vi "TLB Native Dynamic Events ver 0.08b.vi"() -> ()   [LabVIEW 2018]
uses:
  Labview Training Phase 2/Enum Controls/States for Action Engine.ctl
  Type def/TLB event states.ctl
  Type def/TLB MHL States.ctl
  <vilib>/Studica/Studica Toolkit/Background/I2C Channel.ctl
  <vilib>/Studica/Studica Toolkit/NavX/NavX.lvlib
  <vilib>/myRIO/Common/Instrument Driver Framework/myRIO v1.0/AI/typedefs/AI Channels Enum.ctl
  <vilib>/myRIO/Common/Instrument Driver Framework/myRIO v1.0/AI/typedefs/AI Channels List.ctl
  Type def/Type def.ctl
  <vilib>/Studica/Studica Blackhawk/Blackhawk.lvlib
  <vilib>/Studica/Studica Toolkit/Background/Mxp Selection.ctl
  <vilib>/Studica/Studica Toolkit/Background/DIO Channel.ctl
  <vilib>/NI_Real-Time Target Support.lvlib
  <vilib>/ptbypt/NI_PtbyPt.lvlib
  <vilib>/addons/control/pid/NI_PID_pid.lvlib
  Underlying VI's/Webcam FGV Low level ver/State control.ctl
  <vilib>/userdefined/High Color/IMAQdx.ctl
  <vilib>/addons/control/pid/pid.llb/PID (DBL).vi
panel:
  out "Speed and distance cluster":T1
  out "Output":dbl
  in  "SENSOR":bool
  out "Decision":i8
  out "Manual Zero Yaw":bool
  out "Displacement":T2
  out "Fused Heading":dbl
  in  "error in (no error)":errorcluster
  in  "RED LED State":enum16{"OFF", "ON", "BLINK"}(ring)
  in  "GREEN LED State":enum16{"OFF", "ON", "BLINK"}(ring)
  in  "Red LED":bool
  in  "Green LED":bool
  in  "NavX Zero Yaw":bool
  out "Input state":i8
  out "Waveform Chart 2":dbl(graph)
  out "Waveform Chart":dbl(graph)
  in  "STOP":bool
  out "DIO 0":bool
  out "DIO 1":bool
  out "Limit Switch Array":bool[](array[boolean])
  out "error out":errorcluster
  out "L/R average":fxp<+,64,64>
  out "Right Ultrasonic":fxp<+,64,16>
  out "Left Ultrasonic":fxp<+,64,16>
  out "Right IR Sensor":dbl
  out "Left IR Sensor":dbl
  out "Object detection count":T3
  out "Camera error":errorcluster
  in  "Servo Angle":u8(slide) scale=0.0..180.0
  in  "On/Off":bool
  out "Error":errorcluster
  out "element":T4
  out "Action Queue Items":i32
  out "State Logic Queue Items":i32
  out "Action Queues items":string[](array[string])=["Hardware reset", "Software reset", ""]
  out "State logic":T5=enum."Task 2"
  out "Action State":string
  out "Yaw":dbl
  # "TLB FRAMEWORK STATUS"
  # "Camera Status Loop"
  # "Test Programme written by Calvin Loke    Dated: 28 Aug 2019\nTest Programme revised by Dr Alex See   Dated 30 Aug 2019\n\nProgramme version:   TLB Native Dynamic Events ver 0.04b.vi"
  # "Problems now:\nYaw does not work when code is in last state mode\nSlow acceleration due to loop rate?"
  # "Motor Control Loop"
  # "NAVX Control Loop"
  # "Blackhawk status"
  # "Sensor data"
  # "System Health Status Update"
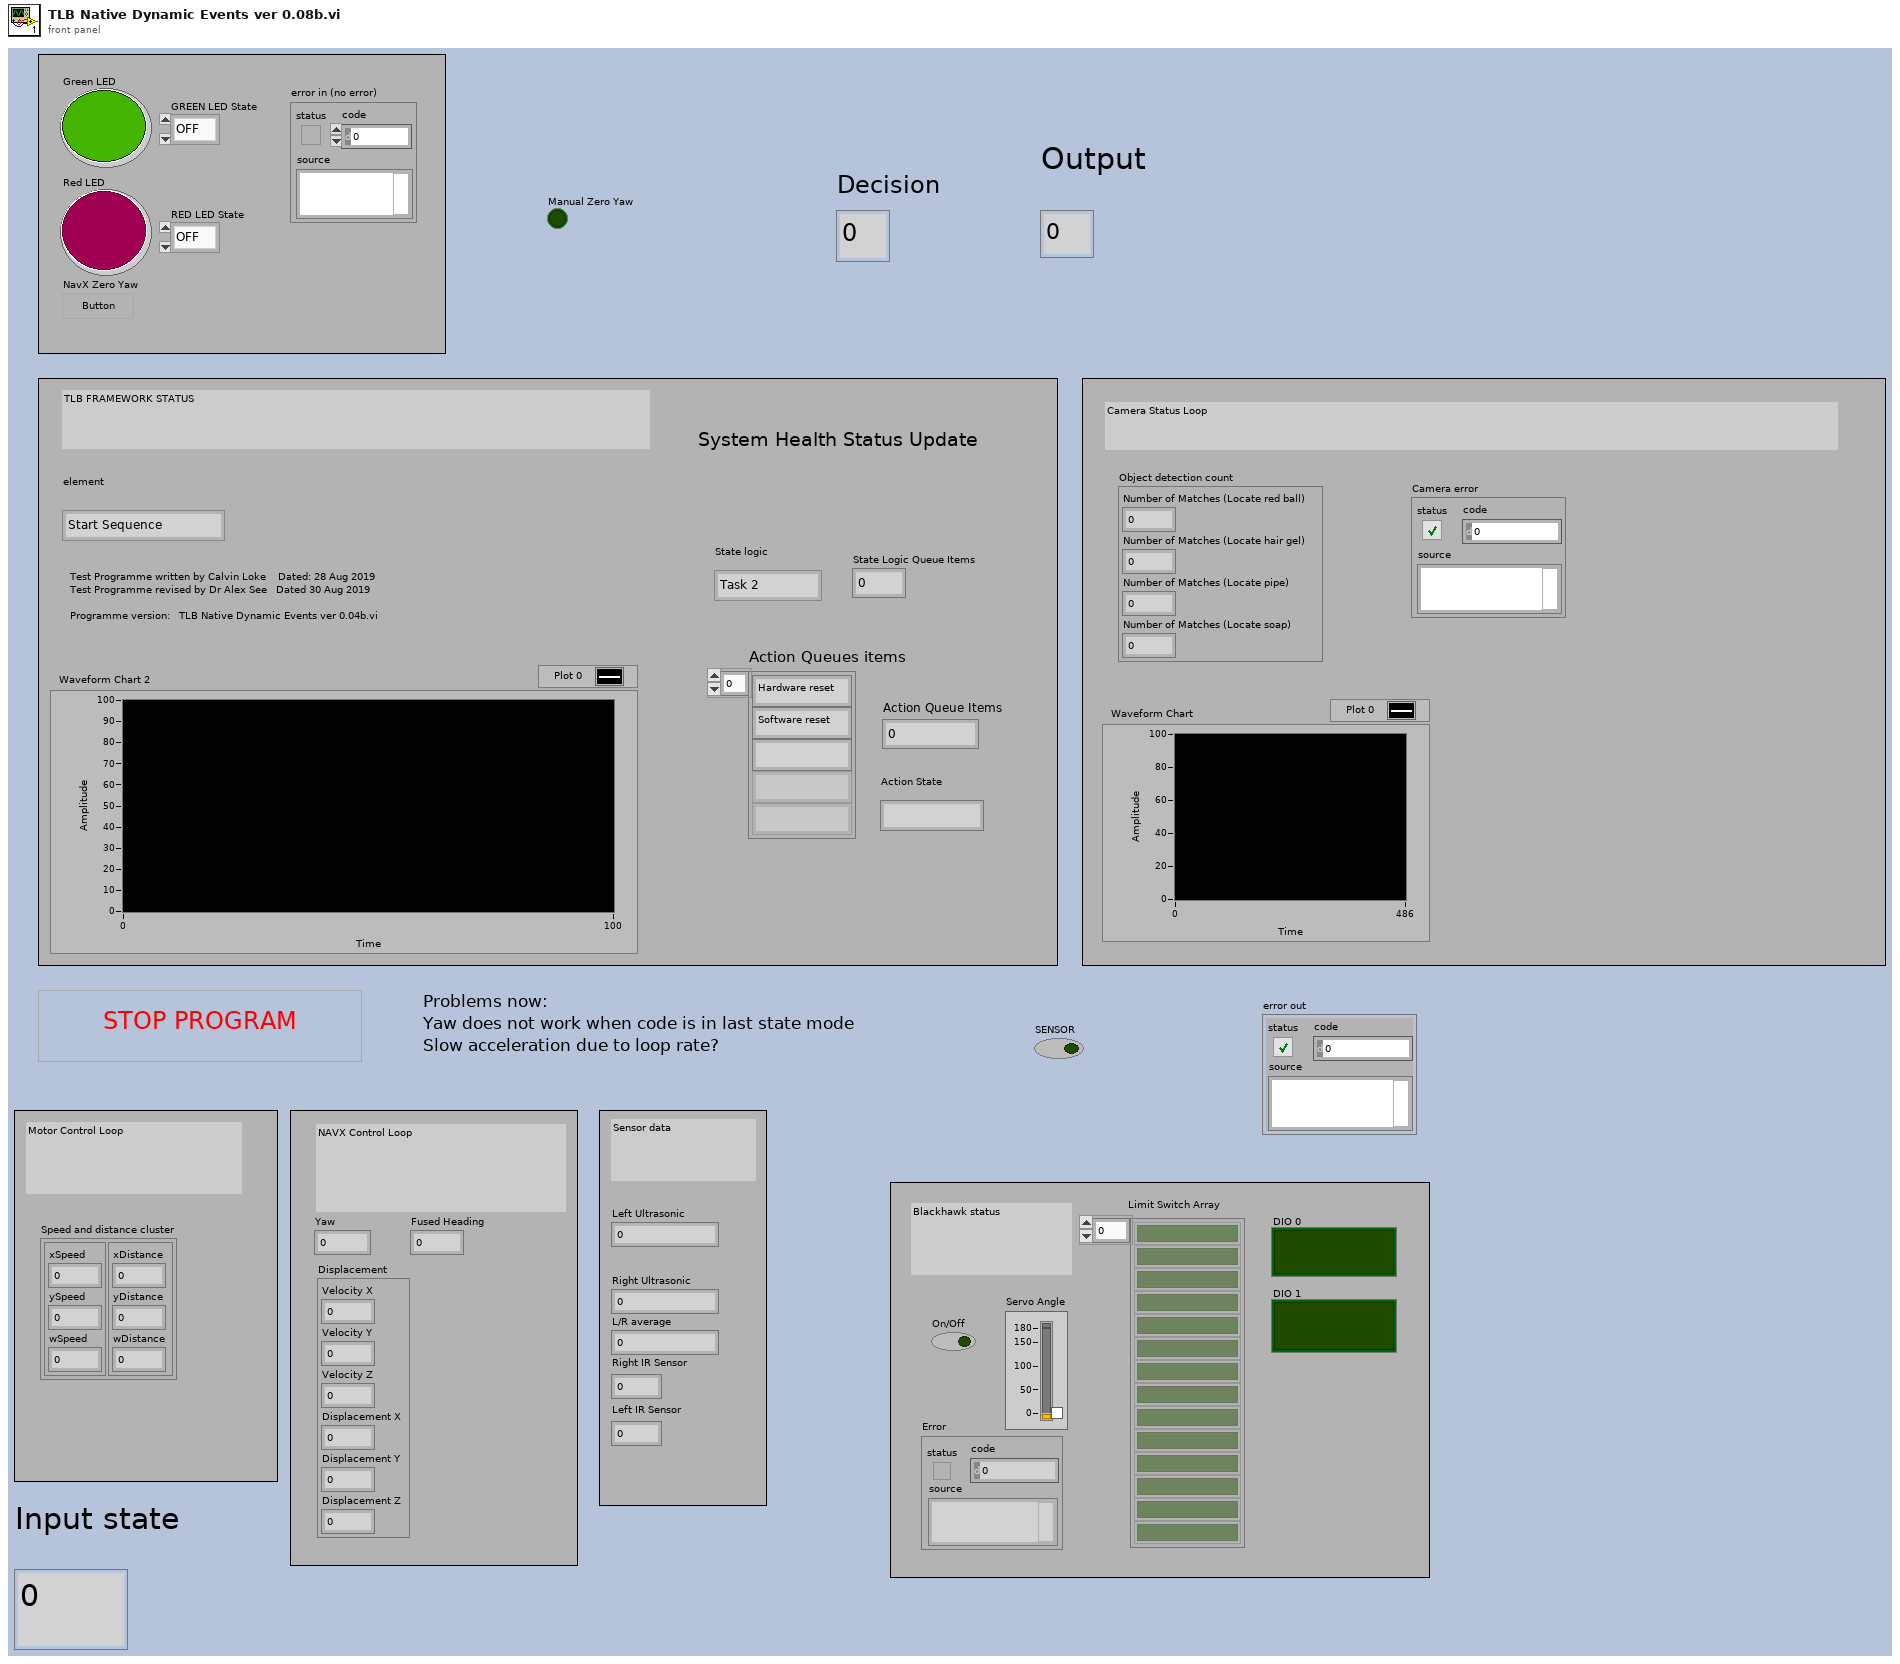
[diagram p1: front panel]
types:
  T1 = cluster{cluster{"xSpeed":dbl, "ySpeed":dbl, "wSpeed":dbl}, cluster{"xDistance":dbl, "yDistance":dbl, "wDistance":dbl}}
  T2 = cluster{"Velocity X":dbl, "Velocity Y":dbl, "Velocity Z":dbl, "Displacement X":dbl, "Displacement Y":dbl, "Displacement Z":dbl}
  T3 = cluster{"Number of Matches (Locate red ball)":i32, "Number of Matches (Locate hair gel)":i32, "Number of Matches (Locate pipe)":i32, "Number of Matches (Locate soap)":i32}
  T4 = typedef "TLB event states.ctl" = enum16{"Start Sequence", "Exit", "Start Task 1", "Start Task 2", "Start Task 3", "Start Task 4", "Camera vision", "Wall follow mode", "Idle", "Start Drive Straight"}
  T5 = typedef "TLB MHL States.ctl" = enum16{"None", "Startup", "Idle", "Processing", "Shutdown", "Reset", "Task 1", "Task 2", "Task 3", "Task 4", "Task 4a", "Task 4b", "Task 4c", "Task 4d", "Task 4e", "Task 4f", "Task 4g", "Task 4h", "Acquire image", "Wall follow mode", "Autodrive", "Autodrive a"}
  T6 = typedef "States for Action Engine.ctl" = enum16{"Initialize", "Write", "Read"}
  T7 = typedef "DIO Channel.ctl" = enum16{"Not Connected", "A/DIO1", "A/DIO2", "A/DIO3", "A/DIO4", "A/DIO5", "A/DIO6", "A/DIO7", "A/DIO13", "B/DIO1", "B/DIO2", "B/DIO3", "B/DIO4", "B/DIO5", "B/DIO6", "B/DIO7", "B/DIO13", "C/DIO0", "C/DIO1", "C/DIO2", "C/DIO3", "C/DIO4", "C/DIO5", "C/DIO6", "C/DIO7"}
  T8 = typedef "Type def.ctl" = cluster{"Front Ultrasonic Obstruct":bool, "Left Ultrasonic Obstruct":bool, "Right Ultrasonic Obstruct ":bool}
  T9 = typedef "I2C Channel.ctl" = enum16{"Not Connected", "A", "B"}
  T10 = enum16{"LAST STATE", "STOP", "FORWARD", "BACKWARD", "LEFT", "RIGHT", "RCW", "ACW", "INIT", "RESET ENCODERS"}
  T11 = cluster{"proportional gain (Kc)":dbl, "integral time (Ti, min)":dbl, "derivative time (Td, min)":dbl}
  T12 = typedef "State control.ctl" = enum16{"Initialise", "Start camera", "Continuous Acquisition ", "Stop camera", "Dispose all"}
  T13 = typedef "IMAQdx.ctl" = refnum<k21>
  T14 = typedef "Mxp Selection.ctl" = enum16{"MXP A", "MXP B"}
  T15 = enum16{"DISTANCE READ", "STOP", "FORWARD", "BACKWARD", "LEFT", "RIGHT", "RCW", "ACW", "INIT", "RESET ENCODERS"}
  T16 = typedef "AI Channels List.ctl" = T17[]
  T17 = typedef "AI Channels Enum.ctl" = enum16{"Not Connected", "AudioIn/Left", "AudioIn/Right", "C/AI0", "C/AI1", "A/AI0", "A/AI1", "A/AI2", "A/AI3", "A/AI4", "A/AI5", "A/AI6", "A/AI7", "B/AI0", "B/AI1", "B/AI2", "B/AI3", "B/AI4", "B/AI5", "B/AI6", "B/AI7", "AI/AI0", "AI/AI1", "AI/AI2", "AI/AI3", "A/AI0 (DIFF)", "A/AI1 (DIFF)", "A/AI2 (DIFF)", "A/AI3 (DIFF)", "B/AI0 (DIFF)", "B/AI1 (DIFF)", "B/AI2 (DIFF)", "B/AI3 (DIFF)"}
  T18 = cluster{"DIO Channel":T7, "FPGA VI Reference Out":refnum<k20>}
  T19 = typedef "Analog Scaling Constants List.ctl" = T20[]
  T20 = typedef "Analog Scaling Constants.ctl" = cluster{"LSB Weight (Volts)":dbl, "Offset (Volts)":dbl, "Signed?":bool}
  T21 = cluster{"Scale Constants Array":T19, "FPGA Reference Out":refnum<k20>, "AI Channel":T16}
  T22 = cluster{"I2C Channel":T9, "FPGA VI Reference Out":refnum<k20>}
  T23 = typedef "NI_Real-Time Target Support.lvlib/RT CPU Load.ctl" = cluster{"Total (%)":dbl, "Time Critical (%)":dbl, "Timed Structures (%)":dbl, "High (%)":dbl, "Above Normal (%)":dbl, "Normal (%)":dbl, "Background (%)":dbl, "Idle (%)":dbl, "ISR (%)":dbl}
  T24 = cluster{"CPU loads[0]":T23, "CPU loads[1]":T23, "CPU loads[2]":T23, "CPU loads[3]":T23, "CPU loads[4]":T23, "CPU loads[5]":T23, "CPU loads[6]":T23, "CPU loads[7]":T23, "CPU loads[8]":T23}
  T25 = cluster{"I2C Ref Out":cluster{"I2C Channel":T9, "FPGA VI Reference Out":refnum<k20>}, "Connected":bool, "Slave Address (7-bit)":u8, "Registry":u8[]}
  T26 = cluster{"Yaw":dbl, "Roll":dbl, "Pitch":dbl, "Heading":dbl, "Fused Heading":dbl}
  T27 = typedef "IMAQ Image.ctl" = refnum<image>
  T28 = cluster{"xDistance":dbl, "yDistance":dbl, "wDistance":dbl}
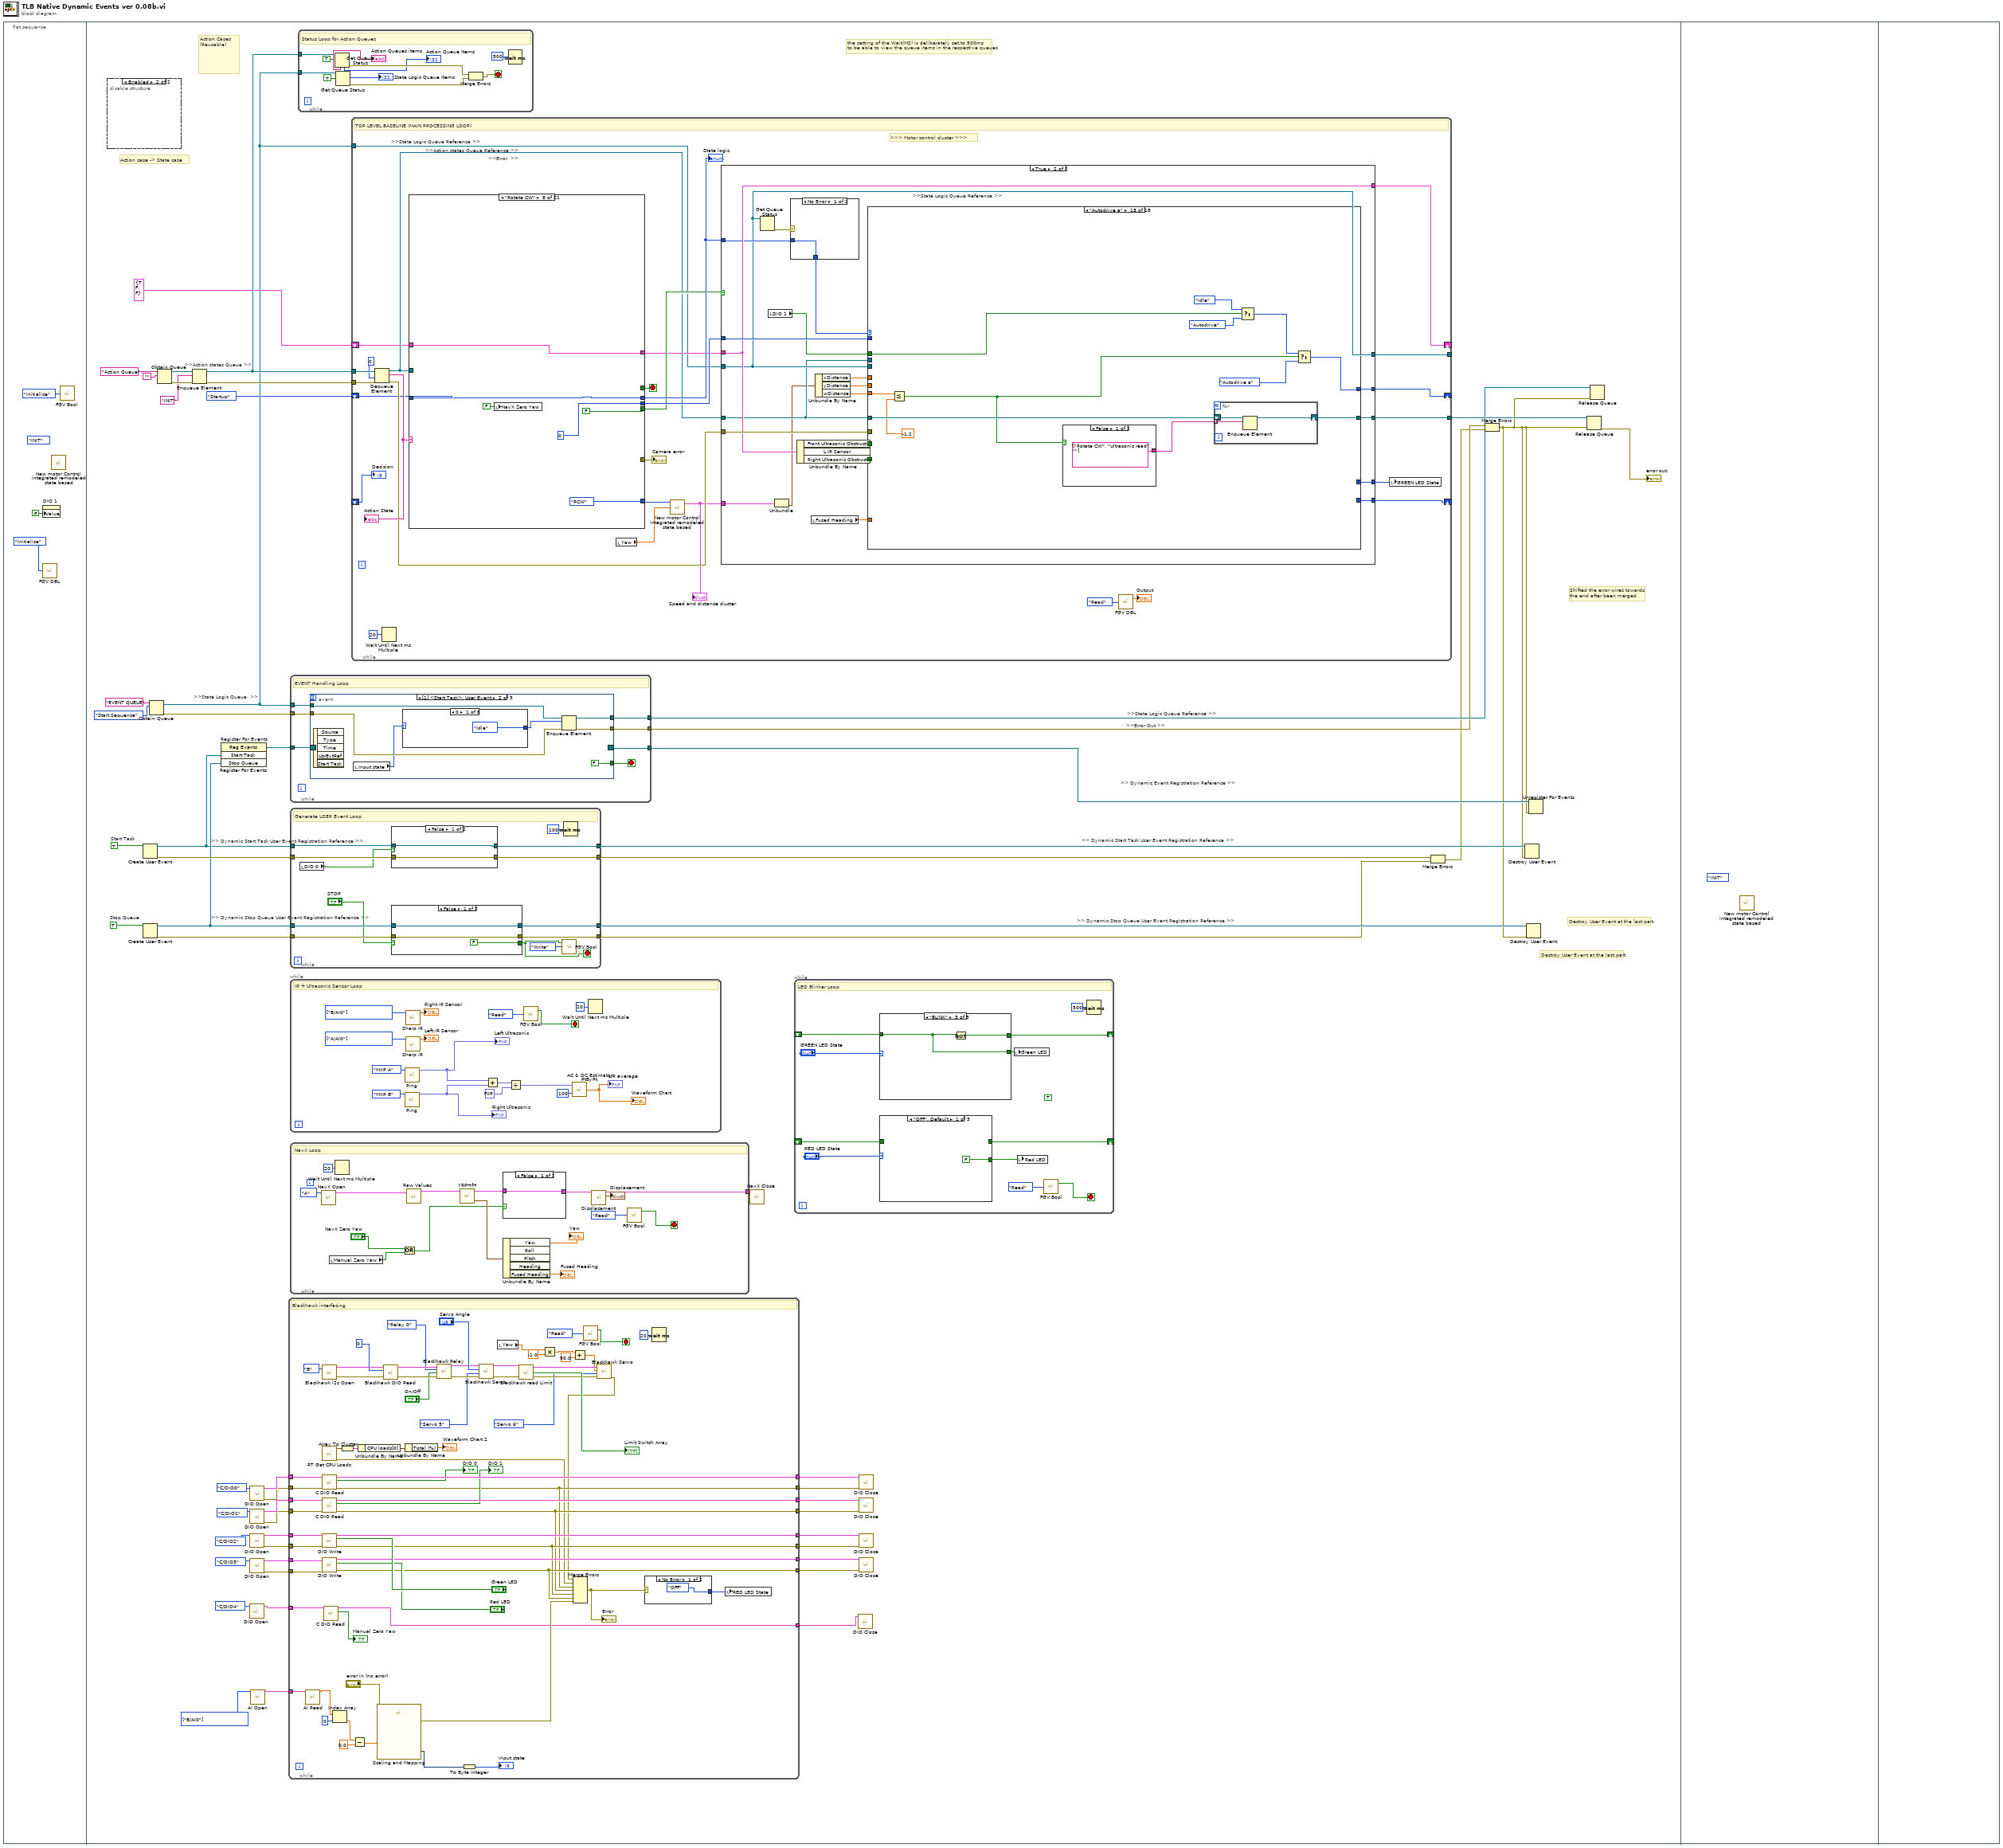
[diagram p0: block diagram]
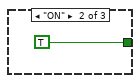
[diagram p2: hidden frame]
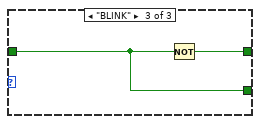
[diagram p3: hidden frame]
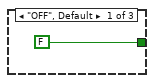
[diagram p4: hidden frame]
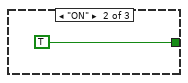
[diagram p5: hidden frame]
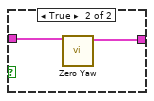
[diagram p6: hidden frame]
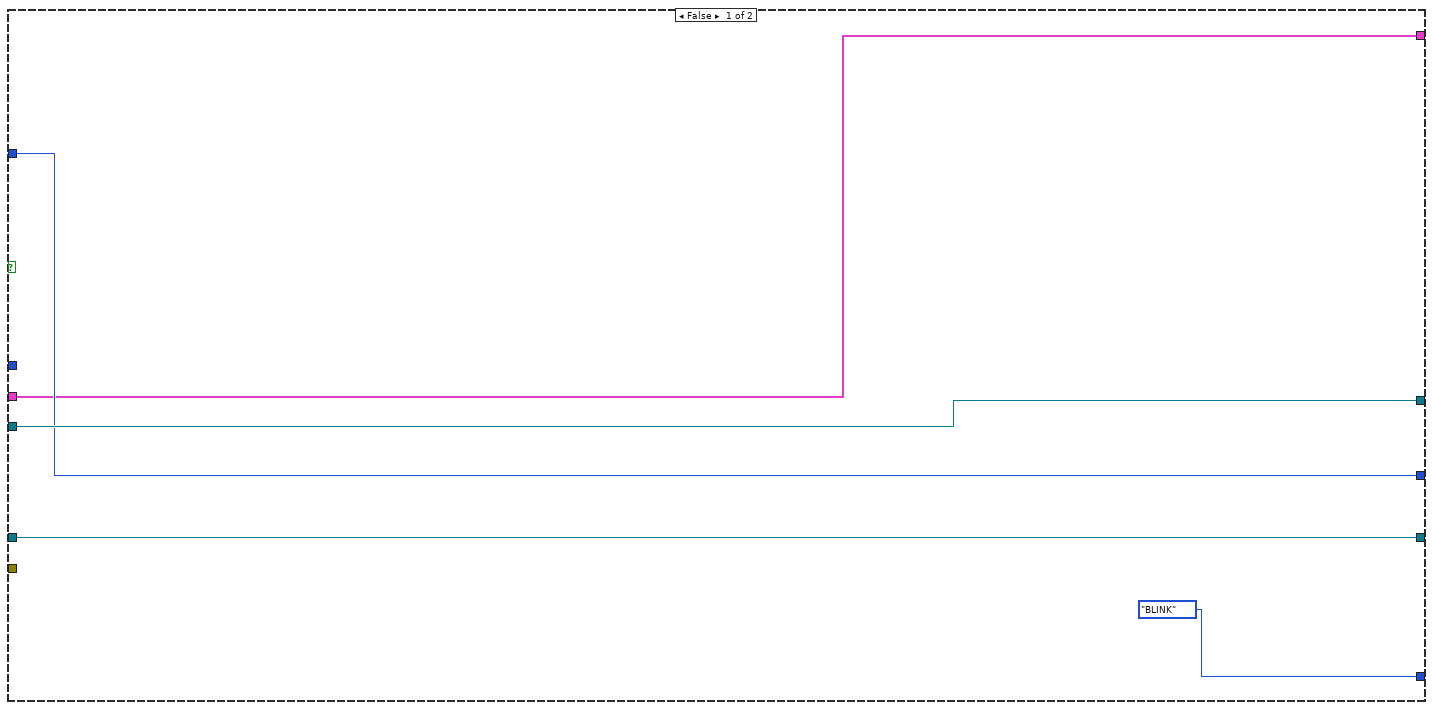
[diagram p7: hidden frame]
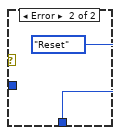
[diagram p8: hidden frame]
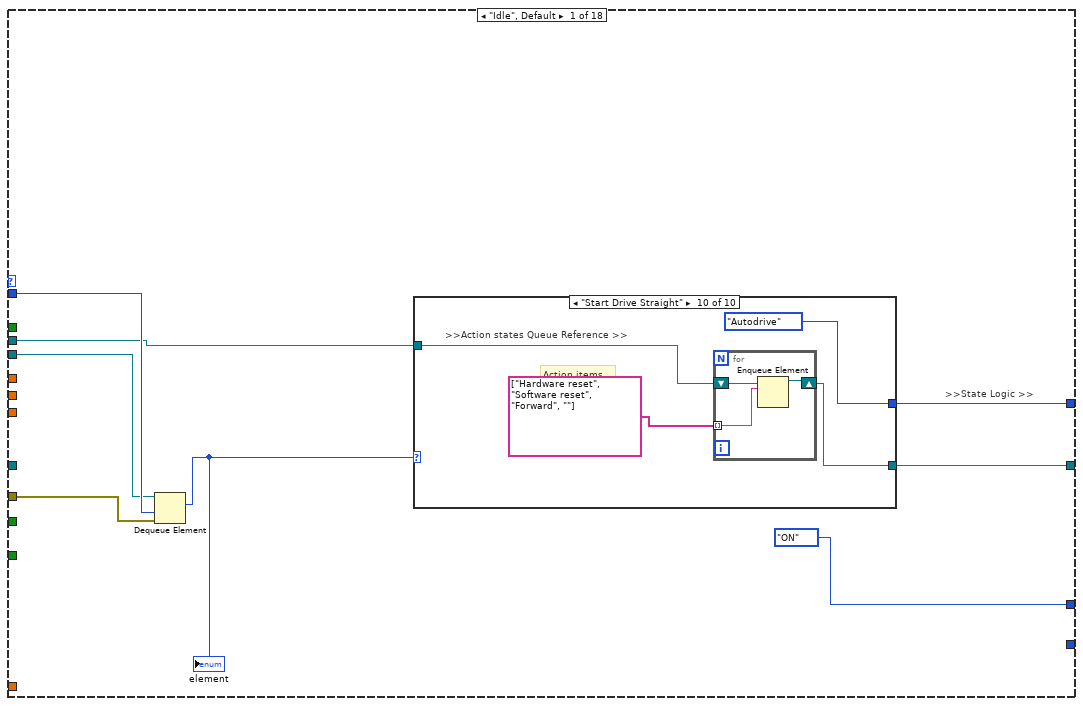
[diagram p9: hidden frame]
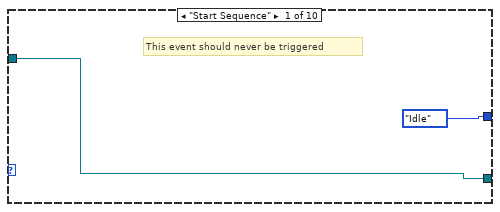
[diagram p10: hidden frame]
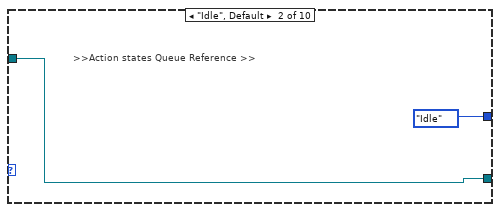
[diagram p11: hidden frame]
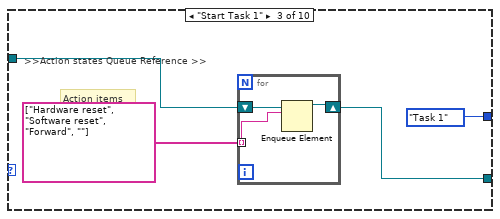
[diagram p12: hidden frame]
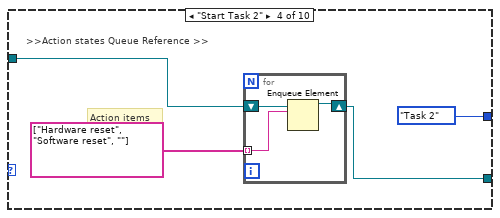
[diagram p13: hidden frame]
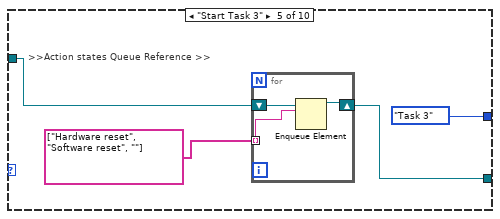
[diagram p14: hidden frame]
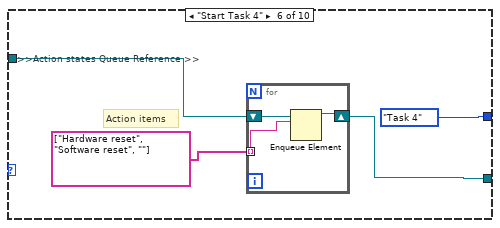
[diagram p15: hidden frame]
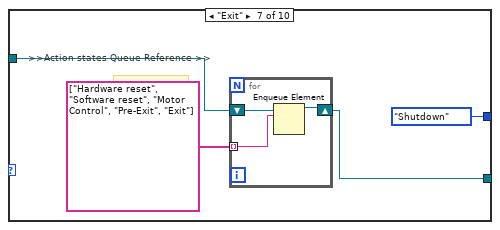
[diagram p16: hidden frame]
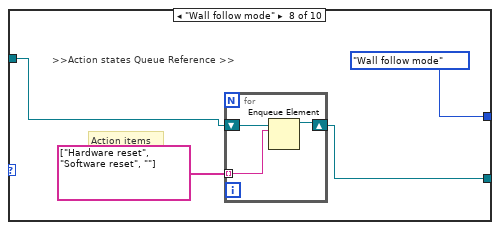
[diagram p17: hidden frame]
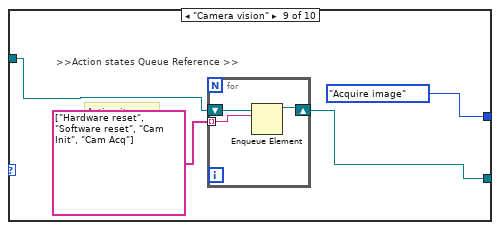
[diagram p18: hidden frame]
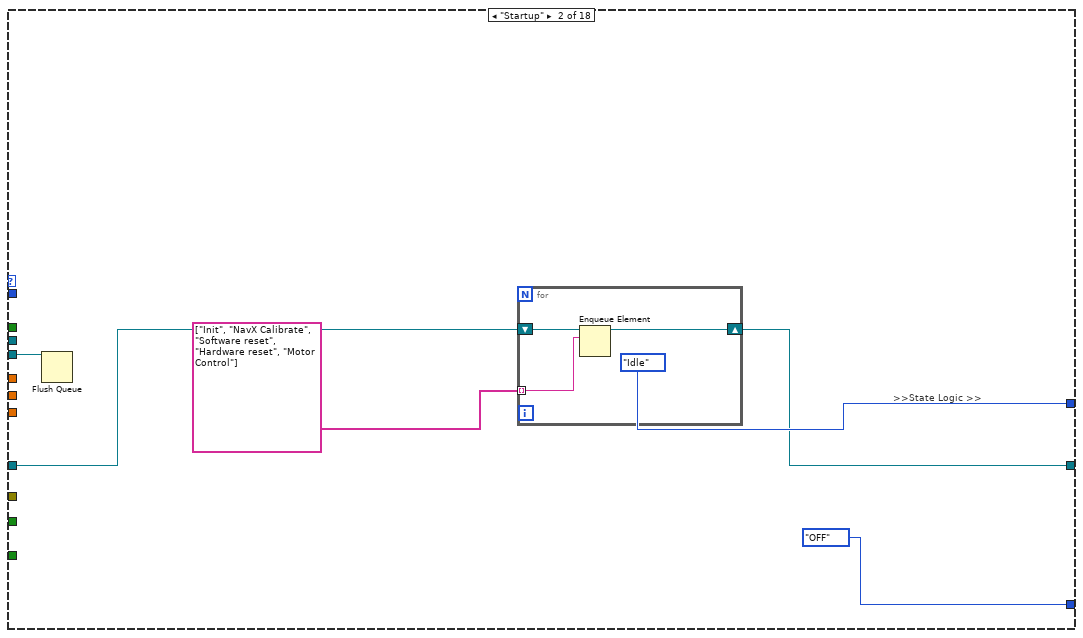
[diagram p19: hidden frame]
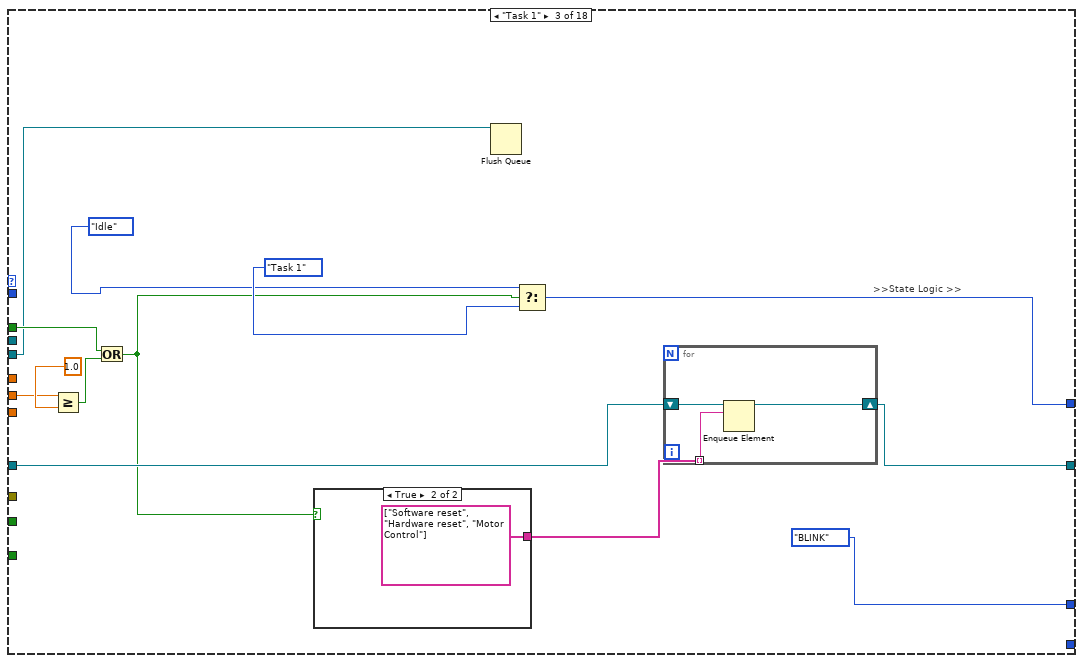
[diagram p20: hidden frame]
diagram:
  n1 = flat-sequence {
    frame #0 {
      (unwired) T15."INIT" ("States")
      n2 = call "FGV DBL.vi"("Init/Read/Write State"=States_for_Action_Engine."Initialize") -> ()  [unwired: 2 in, 2 out]
      n3 = property on="DIO 1" class="Bool (strict)"("Value"=FALSE ("DIO 1")) -> ()  [unwired: 2 in, 2 out]
      n4 = call "New motor Control integrated remodeled state based.vi"() -> ()  [unwired: 3 in, 2 out]
      n5 = call "FGV Bool.vi"("Init/Read/Write State"=States_for_Action_Engine."Initialize") -> ()  [unwired: 2 in, 2 out]
    }
    frame #1 {
      w12 = T16 [enum."B/AI0"] items=["Not Connected", "AudioIn/Left", "AudioIn/Right", "C/AI0", "C/AI1", "A/AI0", "A/AI1", "A/AI2", "A/AI3", "A/AI4", "A/AI5", "A/AI6", "A/AI7", "B/AI0", "B/AI1", "B/AI2", "B/AI3", "B/AI4", "B/AI5", "B/AI6", "B/AI7", "AI/AI0", "AI/AI1", "AI/AI2", "AI/AI3", "A/AI0 (DIFF)", "A/AI1 (DIFF)", "A/AI2 (DIFF)", "A/AI3 (DIFF)", "B/AI0 (DIFF)", "B/AI1 (DIFF)", "B/AI2 (DIFF)", "B/AI3 (DIFF)"] ("AI Channel")
      w60 = TRUE  # Stop Queue
      w59 = TRUE  # Start Task
      # "Action case -> State case"
      # "the setting of the Wait(MS) is deliberately set to 500ms\nto be able to view the queue items in the respective queues"
      # "Action Cases\n(Reusable)"
      # ">>Error Out >>"
      # ">> Dynamic Stop Queue User Event Registration Reference >>"
      # ">> Dynamic Start Task User Event Registration Reference >>"
      # ">> Dynamic Stop Queue User Event Registration Reference >>"
      # ">> Dynamic Start Task User Event Registration Reference >>"
      # ">> Dynamic Event Registration Reference >>"
      # ">>Action states Queue >>"
      # ">>State Logic Queue  >>"
      # ">>State Logic Queue Reference >>"
      # "Destroy User Event at the last part"
      # "Destroy User Event at the last part"
      # "Shifted the error wires towards\nthe end after been merged"
      n6 = disable-structure shown="Enabled" {
        frame Disabled {
          (unwired) variant
          (unwired) TRUE
          n7 = Variant To Data(type="") -> ()  [unwired: 2 in, 2 out]
        }
        frame Enabled {
        }
      }
      n8 = Create User Event(user event datatype=w59) -> (user event=w51:refnum<user-event>, error out=w56:errorcluster)  [unwired: 1 in]
      n9 = Create User Event(user event datatype=w60) -> (user event=w52:refnum<user-event>, error out=w55:errorcluster)  [unwired: 1 in]
      n10 = Obtain Queue(name (unnamed)="EVENT QUEUE", element data type=TLB_event_states."Start Sequence" ("Enum")) -> (queue out=w36:refnum<queue>, error out=w42:errorcluster)  [unwired: 3 in, 1 out]
      n11 = Obtain Queue(name (unnamed)="Action Queue", element data type="") -> (queue out=w45:refnum<queue>, error out=w41:errorcluster)  [unwired: 3 in, 1 out]
      n12 = Enqueue Element(queue=w45, element="INIT", error in (no error)=w41) -> (queue out=w37:refnum<queue>, error out=w40:errorcluster)  [unwired: 1 in, 1 out]
      n13 = register-events "Register For Events"(w51, w52) -> (reference out=w50:refnum<event-registration>)  [unwired: 2 in, 1 out]
      n14 = call <vilib>:"DIO Open.vi"("DIO Channel"=DIO_Channel."C/DIO4") -> ("DIO Info Out"=w6:T18)  [unwired: 9 in, 1 out]
      n15 = call <vilib>:"DIO Open.vi"("DIO Channel"=DIO_Channel."C/DIO0") -> ("error out"=w22:errorcluster, "DIO Info Out"=w28:T18)  [unwired: 9 in]
      n16 = call <vilib>:"DIO Open.vi"("DIO Channel"=DIO_Channel."C/DIO1") -> ("error out"=w20:errorcluster, "DIO Info Out"=w24:T18)  [unwired: 9 in]
      n17 = call <vilib>:"DIO Open.vi"("DIO Channel"=DIO_Channel."C/DIO2") -> ("error out"=w10:errorcluster, "DIO Info Out"=w16:T18)  [unwired: 9 in]
      n18 = call <vilib>:"DIO Open.vi"("DIO Channel"=DIO_Channel."C/DIO3") -> ("error out"=w8:errorcluster, "DIO Info Out"=w15:T18)  [unwired: 9 in]
      n19 = call <vilib>:"AI Open.vi"("AI Channel"=w12) -> ("Analog Info"=w11:T21)  [unwired: 9 in, 1 out]
      n20 = while {
        tunnel: w28 -> [w744]
        tunnel: [w743] -> w27
        tunnel: w24 -> [w742]
        tunnel: [w741] -> w23
        tunnel: w22 -> [w740]
        tunnel: [w709] -> w21
        tunnel: w20 -> [w739]
        tunnel: [w710] -> w19
        tunnel: w16 -> [w733]
        tunnel: w15 -> [w732]
        tunnel: [w729] -> w14
        tunnel: [w728] -> w13
        tunnel: w11 -> [w727]
        tunnel: w10 -> [w720]
        tunnel: [w711] -> w9
        tunnel: w8 -> [w719]
        tunnel: [w712] -> w7
        tunnel: w6 -> [w700]
        tunnel: [w699] -> w4
        stop <- w757 stop-if-true
        # "Blackhawk interfacing"
        n21 = call <vilib>:"AI Read.vi"("Analog Info"=w727) -> ("Array"=w723:dbl[])  [unwired: 9 in, 1 out]
        n22 = call <vilib>:"Blackhawk i2c Open.vi"("I2C Channel"=I2C_Channel."B") -> ("I2C Ref Out"=w735:T22, "error out"=w734:errorcluster)  [unwired: 2 in]
        n23 = call <vilib>:"RT Get CPU Loads.vi"() -> ("error out"=w708:errorcluster, "CPU loads"=w714:T23[])  [unwired: 10 in]
        n24 = call <vilib>:"C DIO Read.vi"("error in (no error)"=w740, "DIO Info In in"=w744) -> ("error out"=w709:errorcluster, "IN"=→"DIO 0":bool, "DIO Info In out"=w743:T18)  [unwired: 7 in]
        n25 = call <vilib>:"C DIO Read.vi"("error in (no error)"=w739, "DIO Info In in"=w742) -> ("error out"=w710:errorcluster, "IN"=→"DIO 1":bool, "DIO Info In out"=w741:T18)  [unwired: 7 in]
        n26 = call <vilib>:"DIO Write.vi"("error in (no error)"=w720, "Input"="Green LED", "DIO Info In"=w733) -> ("error out"=w711:errorcluster, "DIO Info Out"=w729:T18)  [unwired: 7 in]
        n27 = call <vilib>:"DIO Write.vi"("error in (no error)"=w719, "Input"="Red LED", "DIO Info In"=w732) -> ("error out"=w712:errorcluster, "DIO Info Out"=w728:T18)  [unwired: 7 in]
        n28 = call <vilib>:"C DIO Read.vi"("DIO Info In in"=w700) -> ("IN"=→"Manual Zero Yaw":bool, "DIO Info In out"=w699:T18)  [unwired: 8 in, 1 out]
        n29 = Index Array(array=w723, index=0) -> (element=w725:dbl)
        n30 = Array To Cluster(array=w714) -> (cluster=w715:T24)
        n31 = Subtract(x=w725, y=0.0) -> (x-y=w726:dbl)
        n32 = Unbundle By Name(w715) -> ("CPU loads[0]"=w716:T23)
        n33 = call "Scaling and Mapping"("error in (no error)"="error in (no error)", "Signals"=w726) -> ("error out"=w713:errorcluster, "Scaled Signals"=w721:dynamicdata)  [unwired: 8 in]
        n34 = call <vilib>:"Blackhawk DIO Read.vi"("I2C Ref In"=w735, "PIN"=u8 0, "error in (no error)"=w734) -> ("I2C Ref Out"=w755:T22, "error out"=w756:errorcluster)  [unwired: 3 in, 1 out]
        n35 = Unbundle By Name(w716) -> ("Total (%)"=→"Waveform Chart 2":dbl)
        n36 = call <vilib>:"Blackhawk Relay.vi"("error in (no error)"=w756, "On/Off"="On/Off", "Relay"=enum8{"Relay 0", "Relay 1", "Relay 2"}."Relay 0", "I2C Ref In"=w755) -> ("error out"=w752:errorcluster, "I2C Ref Out"=w749:T22)  [unwired: 6 in]
        n37 = To Byte Integer(number=w721) -> (8bit integer=→"Input state":i8)
        n38 = call <vilib>:"Blackhawk Servo.vi"("error in (no error)"=w752, "Servo Select"=enum16{"Servo 5", "Servo 6"}."Servo 5", "Servo Angle"="Servo Angle", "I2C Ref In"=w749) -> ("error out"=w747:errorcluster, "I2C Ref Out"=w746:T22)  [unwired: 6 in]
        n39 = local read "Yaw"() -> (w694:dbl)
        n40 = call <vilib>:"Blackhawk read Limit.vi"("error in (no error)"=w747, "I2C Ref In"=w746) -> ("error out"=w704:errorcluster, "Limit Switch Array"=→"Limit Switch Array":bool[], "I2C Ref Out"=w702:T22)  [unwired: 1 in]
        n41 = Multiply(x=w694, y=-1.0) -> (x*y=w695:dbl)
        n42 = Add(x=w695, y=90.0) -> (x+y=w696:dbl)
        n43 = call "FGV Bool.vi"("Init/Read/Write State"=States_for_Action_Engine."Read") -> ("Output node"=w757:bool)  [unwired: 2 in, 1 out]
        n44 = call <vilib>:"Blackhawk Servo.vi"("error in (no error)"=w704, "Servo Select"=enum16{"Servo 5", "Servo 6"}."Servo 6", "Servo Angle"=w696, "I2C Ref In"=w702) -> ("error out"=w703:errorcluster)  [unwired: 6 in, 1 out]
        n45 = Merge Errors(w703, w708, w709, w710, w711, w712, w713) -> (w707:errorcluster)
        "Error" <- w707
        n46 = case shown="No Error" w707 {
          tunnel: [enum16{"OFF", "ON", "BLINK"}."OFF" ("RED LED State") enum16{"OFF", "ON", "BLINK"}."BLINK" ("RED LED State")] -> w718
          frame No Error {
          }
          frame Error {
          }
        }
        n47 = Wait (ms)(milliseconds to wait=u32 20) -> ()  [unwired: 1 out]
        n48 = local write "RED LED State"(w718) -> ()
      }
      n49 = while {
        tunnel: w50 -> [w637]
        tunnel: [w636] -> w49
        tunnel: w36 -> [w634]
        tunnel: [w633] -> w48
        tunnel: w42 -> [w632]
        tunnel: [w631] -> w39
        stop <- w635 stop-if-true
        # "EVENT Handling Loop"
        n50 = event shown="[1] <Start Task>: User Event" {
          selector: w637 -> [_ _ _]
          dyn-events: [_ _ _] -> w636
          timeout: _ -> [_ _ _]
          tunnel: [FALSE FALSE w664] -> w635
          tunnel: w634 -> [w642 w649 w662]
          tunnel: [w641 w648 w663] -> w633
          tunnel: w632 -> [w639 w647 w660]
          tunnel: [w638 w646 w659] -> w631
          event Timeout {
            n51 = event-data() -> ()  [unwired: 1 in, 3 out]
            n52 = Enqueue Element(queue=w642, element=TLB_event_states."Idle" ("Enum"), error in (no error)=w639) -> (queue out=w641:refnum<queue>, error out=w638:errorcluster)  [unwired: 1 in, 1 out]
          }
          event User Event {
            n53 = event-data() -> ()  [unwired: 1 in, 5 out]
            n54 = local read "Input state"() -> (w645:i8)
            n55 = case shown="0" w645 {
              tunnel: [TLB_event_states."Idle" ("Enum") TLB_event_states."Start Task 1" ("Enum") TLB_event_states."Start Task 2" ("Enum") TLB_event_states."Start Task 3" ("Enum") TLB_event_states."Start Task 4" ("Enum") TLB_event_states."Wall follow mode" ("Enum") TLB_event_states."Camera vision" ("Enum") TLB_event_states."Start Drive Straight" ("Enum")] -> w644
              frame 0 {
              }
              frame 1 {
              }
              frame 2 {
              }
              frame 3, Default {
              }
              frame 4 {
              }
              frame 5 {
              }
              frame 6 {
              }
              frame 7 {
              }
            }
            n56 = Enqueue Element(queue=w649, element=w644, error in (no error)=w647) -> (queue out=w648:refnum<queue>, error out=w646:errorcluster)  [unwired: 1 in, 1 out]
          }
          event User Event {
            n57 = event-data() -> ("Stop Queue"=w664:bool)  [unwired: 1 in, 4 out]
            n58 = Enqueue Element At Opposite End(queue=w662, element=TLB_event_states."Exit" ("Enum"), error in (no error)=w660) -> (queue out=w663:refnum<queue>, error out=w659:errorcluster)  [unwired: 1 in, 1 out]
          }
        }
      }
      n59 = while {
        tunnel: w51 -> [w676]
        tunnel: w52 -> [w675]
        tunnel: [w674] -> w58
        tunnel: [w673] -> w57
        tunnel: w56 -> [w672]
        tunnel: [w671] -> w54
        tunnel: w55 -> [w670]
        tunnel: [w669] -> w53
        stop <- w667 stop-if-true
        # "Generate USER Event Loop"
        n60 = local read "DIO 0"() -> (w666:bool)
        n61 = case shown="False" w666 {
          selector: w666 -> [_ w688]
          tunnel: w676 -> [w687 w692]
          tunnel: [w687 w691] -> w673
          tunnel: w672 -> [w686 w690]
          tunnel: [w686 w689] -> w671
          frame False {
          }
          frame True {
            n62 = Generate User Event(user event=w692, event data cluster=w688, error in=w690) -> (user event out=w691:refnum<user-event>, error out=w689:errorcluster)  [unwired: 1 in]
          }
        }
        n63 = case shown="False" "STOP" {
          selector: "STOP" -> [_ w681]
          tunnel: w675 -> [w680 w685]
          tunnel: [w680 w684] -> w674
          tunnel: w670 -> [w679 w683]
          tunnel: [w679 w682] -> w669
          tunnel: [FALSE w681] -> w667
          frame False {
          }
          frame True {
            n64 = Generate User Event(user event=w685, event data cluster=w681, error in=w683) -> (user event out=w684:refnum<user-event>, error out=w682:errorcluster)  [unwired: 1 in]
          }
        }
        n65 = call "FGV Bool.vi"("Init/Read/Write State"=States_for_Action_Engine."Write", "Input Node"=w667) -> ()  [unwired: 1 in, 2 out]
        n66 = Wait (ms)(milliseconds to wait=u32 100) -> ()  [unwired: 1 out]
      }
      n67 = while {
        stop <- w613 stop-if-true
        w618 = T16 [enum."A/AI0"] items=["Not Connected", "AudioIn/Left", "AudioIn/Right", "C/AI0", "C/AI1", "A/AI0", "A/AI1", "A/AI2", "A/AI3", "A/AI4", "A/AI5", "A/AI6", "A/AI7", "B/AI0", "B/AI1", "B/AI2", "B/AI3", "B/AI4", "B/AI5", "B/AI6", "B/AI7", "AI/AI0", "AI/AI1", "AI/AI2", "AI/AI3", "A/AI0 (DIFF)", "A/AI1 (DIFF)", "A/AI2 (DIFF)", "A/AI3 (DIFF)", "B/AI0 (DIFF)", "B/AI1 (DIFF)", "B/AI2 (DIFF)", "B/AI3 (DIFF)"] ("AI Channel")
        w619 = T16 [enum."B/AI0"] items=["Not Connected", "AudioIn/Left", "AudioIn/Right", "C/AI0", "C/AI1", "A/AI0", "A/AI1", "A/AI2", "A/AI3", "A/AI4", "A/AI5", "A/AI6", "A/AI7", "B/AI0", "B/AI1", "B/AI2", "B/AI3", "B/AI4", "B/AI5", "B/AI6", "B/AI7", "AI/AI0", "AI/AI1", "AI/AI2", "AI/AI3", "A/AI0 (DIFF)", "A/AI1 (DIFF)", "A/AI2 (DIFF)", "A/AI3 (DIFF)", "B/AI0 (DIFF)", "B/AI1 (DIFF)", "B/AI2 (DIFF)", "B/AI3 (DIFF)"] ("AI Channel")
        # "IR + Ultrasonic Sensor Loop"
        n68 = call <vilib>:"Ping.vi"("Mxp Side"=Mxp_Selection."MXP B") -> ("CM"=w607:fxp<+,64,16>)  [unwired: 8 in, 2 out]
        "Right Ultrasonic" <- w607
        n69 = call <vilib>:"Ping.vi"("Mxp Side"=Mxp_Selection."MXP A") -> ("CM"=w608:fxp<+,64,16>)  [unwired: 8 in, 2 out]
        "Left Ultrasonic" <- w608
        n70 = call <vilib>:"Sharp IR.vi"("AI Channel"=w619) -> ("Sharp IR Distance"=→"Right IR Sensor":dbl)  [unwired: 8 in, 2 out]
        n71 = call <vilib>:"Sharp IR.vi"("AI Channel"=w618) -> ("Sharp IR Distance"=→"Left IR Sensor":dbl)  [unwired: 8 in, 2 out]
        n72 = Add(x=w608, y=w607) -> (x+y=w610:fxp<+,64,17>)
        n73 = Divide(x=w610, y=fxp<+,64,17> 2.0) -> (x/y=w606:fxp<+,64,64>)
        n74 = call "FGV Bool.vi"("Init/Read/Write State"=States_for_Action_Engine."Read") -> ("Output node"=w613:bool)  [unwired: 2 in, 1 out]
        n75 = call <vilib>:"AC & DC Estimator PtByPt.vi"("signal"=w606, "sample length"=100) -> ("DC estimate (V)"=→"L/R average" →"Waveform Chart":dbl)  [unwired: 1 in, 2 out]
        n76 = Wait Until Next ms Multiple(millisecond multiple=u32 20) -> ()  [unwired: 1 out]
      }
      n77 = while {
        tunnel: [w86] -> w29
        stop <- w94 stop-if-true
        # "NavX Loop"
        n78 = call <vilib>:"NavX Open.vi"("I2C Channel"=I2C_Channel."A") -> ("NavX Info"=w88:T25)  [unwired: 9 in, 1 out]
        n79 = local read "Manual Zero Yaw"() -> (w82:bool)
        n80 = Wait Until Next ms Multiple(millisecond multiple=u32 20) -> ()  [unwired: 1 out]
        n81 = Or(x="NavX Zero Yaw", y=w82) -> (x .or. y?=w83:bool)
        n82 = call <vilib>:"Raw Values.vi"("NavX Info In"=w88) -> ("NavX Info Out"=w91:T25)  [unwired: 8 in, 1 out]
        n83 = call <vilib>:"YRPHfH.vi"("NavX Info In"=w91) -> ("YRPHfH"=w92:T26, "NavX Info Out"=w90:T25)  [unwired: 3 in]
        n84 = case shown="False" w83 {
          tunnel: [w96 w98] -> w87
          tunnel: w90 -> [w96 w97]
          frame False {
          }
          frame True {
            n85 = call <vilib>:"Zero Yaw.vi"("NavX Info In"=w97) -> ("NavX Info Out"=w98:T25)  [unwired: 10 in]
          }
        }
        n86 = Unbundle By Name(w92) -> ("Yaw"=→"Yaw":dbl, "Fused Heading"=→"Fused Heading":dbl)  [unwired: 3 out]
        n87 = call <vilib>:"Displacement.vi"("NavX Info In"=w87) -> ("Displacement"=→"Displacement":T2, "NavX Info Out"=w86:T25)  [unwired: 9 in]
        n88 = call "FGV Bool.vi"("Init/Read/Write State"=States_for_Action_Engine."Read") -> ("Output node"=w94:bool)  [unwired: 2 in, 1 out]
      }
      n89 = while {
        tunnel: w37 -> [w628]
        tunnel: w36 -> [w625]
        stop <- w622 stop-if-true
        # "Status Loop for Action Queues"
        n90 = Get Queue Status(queue=w628, return elements? (F)=TRUE) -> (error out=w624:errorcluster, # elements in queue=→"Action Queue Items":i32, elements=→"Action Queues items":string[])  [unwired: 1 in, 5 out]
        n91 = Get Queue Status(queue=w625, return elements? (F)=TRUE) -> (# pending remove=→"State Logic Queue Items":i32, error out=w623:errorcluster)  [unwired: 1 in, 6 out]
        n92 = Merge Errors(w624, w623) -> (w622:errorcluster)
        n93 = Wait (ms)(milliseconds to wait=u32 500) -> ()  [unwired: 1 out]
      }
      n94 = while {
        tunnel: w36 -> [w109]
        shift-right: [w120] -> _
        shift-left: TLB_MHL_States."Startup" ("Enum") -> [w114]
        tunnel: w37 -> [w125]
        tunnel: w40 -> [w123]
        tunnel: [w122] -> _
        tunnel: [w121] -> w32
        shift-right: [w111] -> _
        shift-left: T8 {"Front Ultrasonic Obstruct"=TRUE, "Left Ultrasonic Obstruct"=FALSE, "Right Ultrasonic Obstruct "=FALSE} -> [w113]
        shift-right: [w102] -> _
        shift-left: _ -> [w101]
        stop <- w107 stop-if-true
        # ">>> Motor control cluster >>>"
        # ">>Error  >>"
        # ">>Action states Queue Reference >>"
        # ">>State Logic Queue Reference >>"
        # "TOP LEVEL BASELINE (MAIN PROCESSING LOOP)"
        n95 = Dequeue Element(queue=w125, timeout in ms (-1)=0, error in (no error)=w123) -> (queue out=w115:refnum<queue>, element=w124:string, error out=w116:errorcluster)  [unwired: 1 out]
        "Action State" <- w124
        n96 = Wait Until Next ms Multiple(millisecond multiple=u32 20) -> ()  [unwired: 1 out]
        n97 = case shown="\"Rotate CW\"" w124 {
          tunnel: [w452 w467 w474 w479 w485 w492 w498 w502 w510 w515 w524 w531 TLB_MHL_States."Shutdown" ("Enum") w541 w552 w555 w566 w577 w585 w597 w601] -> w126
          tunnel: [w455 0 0 0 0 0 0 0 0 0 0 0 0 0 0 0 0 0 0 0 0] -> w119
          tunnel: [TRUE FALSE FALSE FALSE FALSE FALSE FALSE FALSE FALSE FALSE FALSE FALSE FALSE FALSE FALSE FALSE FALSE FALSE FALSE FALSE FALSE] -> w118
          tunnel: w115 -> [_ _ _ _ _ _ _ _ _ _ _ _ _ _ _ _ _ _ _ _ _]
          tunnel: w114 -> [w452 w467 w474 w479 w485 w492 w498 w502 w510 w515 w524 w531 _ w541 w552 w555 w566 w577 w585 w597 w601]
          tunnel: w113 -> [w453 w462 w470 w480 w482 w488 w494 w500 w506 w512 w521 w527 w534 w542 w551 w558 w567 w578 w584 w594 w602]
          tunnel: [w453 w461 w469 w480 w482 w488 w494 w500 w506 w512 w520 w527 w534 w542 w548 w557 w567 w578 w584 w594 w602] -> w112
          tunnel: [_ _ _ _ _ _ _ _ _ _ _ _ _ _ _ _ _ w568 w580 w588 _] -> w110
          tunnel: [_ _ _ _ _ _ _ _ _ _ _ _ TRUE _ _ _ _ _ _ _ _] -> w107
          tunnel: [T10."LAST STATE" ("Move mode") T10."INIT" ("Move mode") T10."FORWARD" ("Move mode") T10."LAST STATE" ("Move mode") T10."BACKWARD" ("Move mode") T10."RIGHT" ("Move mode") T10."LEFT" ("Move mode") T10."RCW" ("Move mode") T10."ACW" ("Move mode") T10."STOP" ("Move mode") _ T10."RESET ENCODERS" ("Move mode") T10."INIT" ("Move mode") T10."INIT" ("Move mode") _ _ _ _ _ _ _] -> w105
          frame "No action", Default {
            n98 = case shown="\"Startup\", Default" w452 {
              tunnel: [0 100] -> w455
              frame "Startup", Default {
              }
              frame "Idle" {
              }
            }
            n99 = local write "NavX Zero Yaw"(FALSE ("NavX Zero Yaw")) -> ()
          }
          frame "Init" {
            # ">>State Logic  >>"
            n100 = local write "Servo Angle"(u8 90 ("Servo Angle")) -> ()
            n101 = Bundle By Name(cluster=w462, "Front Ultrasonic Obstruct"=FALSE ("Object detected"), "L IR Sensor"=0.0, "Right Ultrasonic Obstruct"=FALSE ("In move state?")) -> (w461:T8)
          }
          frame "Forward" {
            n102 = local write "NavX Zero Yaw"(FALSE ("NavX Zero Yaw")) -> ()
            n103 = Bundle By Name(cluster=w470, "Right Ultrasonic Obstruct"=TRUE ("In move state?")) -> (w469:T8)
          }
          frame " Motor Control" {
          }
          frame "Reverse" {
            n104 = local write "NavX Zero Yaw"(FALSE ("NavX Zero Yaw")) -> ()
          }
          frame "Right" {
            n105 = local write "NavX Zero Yaw"(FALSE ("NavX Zero Yaw")) -> ()
          }
          frame "Left" {
            n106 = local write "NavX Zero Yaw"(FALSE ("NavX Zero Yaw")) -> ()
          }
          frame "Rotate CW" {
            n107 = local write "NavX Zero Yaw"(FALSE ("NavX Zero Yaw")) -> ()
          }
          frame "Rotate ACW" {
            n108 = local write "NavX Zero Yaw"(FALSE ("NavX Zero Yaw")) -> ()
          }
          frame "Stop" {
            n109 = local write "NavX Zero Yaw"(FALSE ("NavX Zero Yaw")) -> ()
          }
          frame "Software reset" {
            w517 = FALSE ("NavX Zero Yaw")
            n110 = Wait (ms)(milliseconds to wait=u32 20) -> ()  [unwired: 1 out]
            n111 = local write "NavX Zero Yaw"(w517) -> ()
            n112 = Bundle By Name(cluster=w521, "Front Ultrasonic Obstruct"=w517, "L IR Sensor"=0.0, "Right Ultrasonic Obstruct"=w517) -> (w520:T8)
          }
          frame "Hardware reset" {
            n113 = Wait (ms)(milliseconds to wait=u32 100) -> ()  [unwired: 1 out]
            n114 = local write "NavX Zero Yaw"(TRUE ("NavX Zero Yaw")) -> ()
          }
          frame "Exit" {
          }
          frame "Pre-Exit" {
          }
          frame "Ultrasonic read" {
            # "Object detection"
            n115 = local read "L/R average"() -> (w546:fxp<+,64,64>)
            n116 = Less Or Equal?(x=w546, y=35.0) -> (x <= y?=w545:bool)
            n117 = Or(x=w545, y="SENSOR") -> (x .or. y?=w544:bool)
            n118 = Bundle By Name(cluster=w551, "Front Ultrasonic Obstruct"=w544) -> (w548:T8)
          }
          frame "IR Sensor Read" {
            n119 = local read "Left IR Sensor"() -> (w556:dbl)
            n120 = Bundle By Name(cluster=w558, "L IR Sensor"=w556) -> (w557:T8)
          }
          frame "Calculate" {
            n121 = Unbundle By Name(w567) -> ("L IR Sensor"=w562:dbl)
            n122 = call-poly <vilib>:"PID.vi"("output range"=cluster{"output high":dbl, "output low":dbl} {"output high"=0.3, "output low"=-0.3}, "PID gains"=T11 {"proportional gain (Kc)"=0.01, "integral time (Ti, min)"=0.0, "derivative time (Td, min)"=0.0}, "process variable"=w562, "setpoint"=20.0) -> ("output"=w559:dbl)  [unwired: 6 in, 1 out]
            n123 = Negate(x=w559) -> ()  [unwired: 1 out]
          }
          frame "Cam Init" {
            n124 = call "Low-Level Grab.vi"("States"=State_control."Initialise", "Session In"=T13 "cam1") -> ("error out"=w569:errorcluster, "Session Out"=w570:T13)  [unwired: 7 in, 1 out]
            n125 = call "Low-Level Grab.vi"("error in (no error)"=w569, "States"=State_control."Start camera", "Session In"=w570) -> ("error out"=w568:errorcluster)  [unwired: 6 in, 2 out]
            n126 = local write "Servo Angle"(u8 170 ("Servo Angle")) -> ()
          }
          frame "Cam Acq" {
            n127 = call "Low-Level Grab.vi"("States"=State_control."Continuous Acquisition ") -> ("error out"=w581:errorcluster, "Image Out"=w582:T27)  [unwired: 8 in, 1 out]
            n128 = call "All object detection ver2.vi"("Image In"=w582, "error in"=w581) -> ("Object detection count"=→"Object detection count":T3, "error out"=w580:errorcluster)  [unwired: 1 out]
          }
          frame "Cam Exit" {
            n129 = call "Low-Level Grab.vi"("States"=State_control."Stop camera") -> ("error out"=w589:errorcluster, "Session Out"=w591:T13)  [unwired: 8 in, 1 out]
            n130 = local write "Servo Angle"(u8 90 ("Servo Angle")) -> ()
            n131 = call "Low-Level Grab.vi"("error in (no error)"=w589, "States"=State_control."Dispose all", "Session In"=w591) -> ("error out"=w588:errorcluster)  [unwired: 6 in, 2 out]
          }
          frame "NavX Calibrate" {
            # "Adds a 15 second delay to the startup process \nfor the NavX to calibrate"
            n132 = Wait (ms)(milliseconds to wait=u32 15000) -> ()  [unwired: 1 out]
          }
        }
        "State logic" <- w126
        "Camera error" <- w110
        n133 = local read "Yaw"() -> (w103:dbl)
        n134 = call "New motor Control integrated remodeled state based.vi"("Yaw"=w103, "States"=w105) -> ("Speed and distance cluster"=w104:T1)  [unwired: 1 in, 1 out]
        "Speed and distance cluster" <- w104
        n135 = case shown="True" w118 {
          tunnel: w126 -> [w130 w141]
          tunnel: w109 -> [w131 w140]
          tunnel: w115 -> [w129 w136]
          tunnel: [w131 w140] -> w122
          tunnel: [w129 w152] -> w121
          tunnel: [w130 w151] -> w120
          tunnel: w116 -> [_ w150]
          tunnel: w119 -> [_ w149]
          tunnel: w112 -> [w128 w143]
          tunnel: [w128 w143] -> w111
          tunnel: [enum16{"OFF", "ON", "BLINK"}."BLINK" ("GREEN LED State") w137] -> w106
          tunnel: w104 -> [_ w134]
          tunnel: [_ w132] -> w102
          frame False {
          }
          frame True {
            # ">>State Logic Queue Reference >>"
            n136 = Get Queue Status(queue=w140) -> (error out=w139:errorcluster)  [unwired: 2 in, 7 out]
            n137 = local read "DIO 1"() -> (w138:bool)
            n138 = Unbundle(w134) -> (w133:T28)  [unwired: 1 out]
            n139 = case shown="No Error" w139 {
              tunnel: [w153 TLB_MHL_States."Reset" ("Enum")] -> w142
              tunnel: w141 -> [w153 _]
              frame No Error {
              }
              frame Error {
              }
            }
            n140 = Unbundle By Name(w143) -> ("Front Ultrasonic Obstruct"=w144:bool, "Right Ultrasonic Obstruct"=w135:bool)  [unwired: 1 out]
            n141 = local read "Fused Heading"() -> (w145:dbl)
            n142 = Unbundle By Name(w133) -> ("xDistance"=w146:dbl, "yDistance"=w148:dbl, "wDistance"=w147:dbl)
            n143 = case shown="\"Autodrive a\"" w142 {
              tunnel: w140 -> [w158 w223 w234 w251 w270 w286 w301 w317 w333 w349 _ w373 w395 w408 _ _ _ _]
              tunnel: w136 -> [_ w226 w240 w255 w279 w290 w306 w323 w338 w355 w366 w376 w396 w412 w421 w425 w431 w443]
              tunnel: [w155 w225 w239 w256 w278 w291 w305 w322 w337 w354 w365 w377 w397 w411 w421 w424 w431 w444] -> w152
              tunnel: [w161 TLB_MHL_States."Idle" ("Enum") w242 w257 w275 w294 w308 w321 w339 w353 TLB_MHL_States."Shutdown" ("Enum") w379 w388 w410 TLB_MHL_States."Reset" ("Enum") TLB_MHL_States."Shutdown" ("Enum") TLB_MHL_States."Reset" ("Enum") w438] -> w151
              tunnel: w150 -> [w159 _ _ _ _ _ _ _ _ _ _ _ _ _ _ _ _ _]
              tunnel: w149 -> [w160 _ _ _ _ _ _ _ _ _ _ _ _ _ _ _ _ _]
              tunnel: w138 -> [_ _ w237 w254 w273 _ _ _ _ w352 _ w374 w391 w409 _ _ _ w433]
              tunnel: w148 -> [_ _ w232 _ _ _ w300 w316 _ _ _ _ _ _ _ _ _ _]
              tunnel: w147 -> [_ _ _ _ _ _ _ _ _ _ _ _ _ _ _ _ _ w441]
              tunnel: w146 -> [_ _ _ _ _ _ _ _ w332 _ _ _ _ _ _ _ _ _]
              tunnel: w145 -> [_ _ _ _ w269 _ _ _ _ _ _ _ _ _ _ _ _ _]
              tunnel: w144 -> [_ _ _ w252 _ w288 _ _ _ w351 _ _ w390 _ _ _ _ _]
              tunnel: [enum16{"OFF", "ON", "BLINK"}."ON" ("GREEN LED State") enum16{"OFF", "ON", "BLINK"}."OFF" ("GREEN LED State") enum16{"OFF", "ON", "BLINK"}."BLINK" ("GREEN LED State") enum16{"OFF", "ON", "BLINK"}."BLINK" ("GREEN LED State") enum16{"OFF", "ON", "BLINK"}."BLINK" ("GREEN LED State") enum16{"OFF", "ON", "BLINK"}."BLINK" ("GREEN LED State") enum16{"OFF", "ON", "BLINK"}."BLINK" ("GREEN LED State") enum16{"OFF", "ON", "BLINK"}."BLINK" ("GREEN LED State") enum16{"OFF", "ON", "BLINK"}."BLINK" ("GREEN LED State") enum16{"OFF", "ON", "BLINK"}."BLINK" ("GREEN LED State") enum16{"OFF", "ON", "BLINK"}."OFF" ("GREEN LED State") enum16{"OFF", "ON", "BLINK"}."BLINK" ("GREEN LED State") enum16{"OFF", "ON", "BLINK"}."BLINK" ("GREEN LED State") enum16{"OFF", "ON", "BLINK"}."BLINK" ("GREEN LED State") _ enum16{"OFF", "ON", "BLINK"}."OFF" ("GREEN LED State") _ _] -> w137
              tunnel: w136 -> [w156 _ _ _ _ _ _ _ _ _ _ _ _ _ _ _ _ _]
              tunnel: w135 -> [_ _ _ _ _ _ _ _ _ _ _ _ _ _ _ _ _ _]
              tunnel: [_ _ _ _ _ _ _ _ _ _ _ _ w386 _ _ _ _ _] -> w132
              frame "Idle", Default {
                # ">>State Logic >>"
                n144 = Dequeue Element(queue=w158, timeout in ms (-1)=w160, error in (no error)=w159) -> (element=w162:T4)  [unwired: 3 out]
                "element" <- w162
                n145 = case shown="\"Start Drive Straight\"" w162 {
                  tunnel: [TLB_MHL_States."Idle" ("Enum") TLB_MHL_States."Idle" ("Enum") TLB_MHL_States."Task 1" ("Enum") TLB_MHL_States."Task 2" ("Enum") TLB_MHL_States."Task 3" ("Enum") TLB_MHL_States."Task 4" ("Enum") TLB_MHL_States."Shutdown" ("Enum") TLB_MHL_States."Wall follow mode" ("Enum") TLB_MHL_States."Acquire image" ("Enum") TLB_MHL_States."Autodrive" ("Enum")] -> w161
                  tunnel: w156 -> [w163 w165 w169 w176 w182 w190 w197 w204 w211 w218]
                  tunnel: [w163 w165 w168 w175 w183 w189 w196 w203 w210 w216] -> w155
                  frame "Start Sequence" {
                    # "This event should never be triggered"
                  }
                  frame "Idle", Default {
                    # ">>Action states Queue Reference >>"
                  }
                  frame "Start Task 1" {
                    # ">>Action states Queue Reference >>"
                    # "Action items"
                    n146 = for {
                      shift-right: [w173] -> w168
                      shift-left: w169 -> [w172]
                      tunnel: string[] ["Hardware reset", "Software reset", "Forward", ""] -> [w171] mode=indexing
                      n147 = Enqueue Element(queue=w172, element=w171) -> (queue out=w173:refnum<queue>)  [unwired: 2 in, 2 out]
                    }
                  }
                  frame "Start Task 2" {
                    # ">>Action states Queue Reference >>"
                    # "Action items"
                    n148 = for {
                      shift-right: [w180] -> w175
                      shift-left: w176 -> [w179]
                      tunnel: string[] ["Hardware reset", "Software reset", ""] -> [w178] mode=indexing
                      n149 = Enqueue Element(queue=w179, element=w178) -> (queue out=w180:refnum<queue>)  [unwired: 2 in, 2 out]
                    }
                  }
                  frame "Start Task 3" {
                    # ">>Action states Queue Reference >>"
                    n150 = for {
                      shift-right: [w187] -> w183
                      shift-left: w182 -> [w186]
                      tunnel: string[] ["Hardware reset", "Software reset", ""] -> [w185] mode=indexing
                      n151 = Enqueue Element(queue=w186, element=w185) -> (queue out=w187:refnum<queue>)  [unwired: 2 in, 2 out]
                    }
                  }
                  frame "Start Task 4" {
                    # ">>Action states Queue Reference >>"
                    # "Action items"
                    n152 = for {
                      shift-right: [w194] -> w189
                      shift-left: w190 -> [w193]
                      tunnel: string[] ["Hardware reset", "Software reset", ""] -> [w192] mode=indexing
                      n153 = Enqueue Element(queue=w193, element=w192) -> (queue out=w194:refnum<queue>)  [unwired: 2 in, 2 out]
                    }
                  }
                  frame "Exit" {
                    # ">>Action states Queue Reference >>"
                    # "Action items"
                    n154 = for {
                      shift-right: [w201] -> w196
                      shift-left: w197 -> [w200]
                      tunnel: string[] ["Hardware reset", "Software reset", "Motor Control", "Pre-Exit", "Exit"] -> [w199] mode=indexing
                      n155 = Enqueue Element(queue=w200, element=w199) -> (queue out=w201:refnum<queue>)  [unwired: 2 in, 2 out]
                    }
                  }
                  frame "Wall follow mode" {
                    # ">>Action states Queue Reference >>"
                    # "Action items"
                    n156 = for {
                      shift-right: [w208] -> w203
                      shift-left: w204 -> [w207]
                      tunnel: string[] ["Hardware reset", "Software reset", ""] -> [w206] mode=indexing
                      n157 = Enqueue Element(queue=w207, element=w206) -> (queue out=w208:refnum<queue>)  [unwired: 2 in, 2 out]
                    }
                  }
                  frame "Camera vision" {
                    # ">>Action states Queue Reference >>"
                    # "Action items"
                    n158 = for {
                      shift-right: [w215] -> w210
                      shift-left: w211 -> [w214]
                      tunnel: string[] ["Hardware reset", "Software reset", "Cam Init", "Cam Acq"] -> [w213] mode=indexing
                      n159 = Enqueue Element(queue=w214, element=w213) -> (queue out=w215:refnum<queue>)  [unwired: 2 in, 2 out]
                    }
                  }
                  frame "Start Drive Straight" {
                    # ">>Action states Queue Reference >>"
                    # "Action items"
                    n160 = for {
                      shift-right: [w222] -> w216
                      shift-left: w218 -> [w221]
                      tunnel: string[] ["Hardware reset", "Software reset", "Forward", ""] -> [w220] mode=indexing
                      n161 = Enqueue Element(queue=w221, element=w220) -> (queue out=w222:refnum<queue>)  [unwired: 2 in, 2 out]
                    }
                  }
                }
              }
              frame "Startup" {
                # ">>State Logic >>"
                n162 = Flush Queue(queue=w223) -> ()  [unwired: 1 in, 3 out]
                n163 = for {
                  shift-right: [w230] -> w225
                  shift-left: w226 -> [w231]
                  tunnel: string[] ["Init", "NavX Calibrate", "Software reset", "Hardware reset", "Motor Control"] -> [w229] mode=indexing
                  n164 = Enqueue Element(queue=w231, element=w229) -> (queue out=w230:refnum<queue>)  [unwired: 2 in, 2 out]
                }
              }
              frame "Task 1" {
                # ">>State Logic >>"
                n165 = Greater Or Equal?(x=w232, y=1.0) -> (x >= y?=w235:bool)
                n166 = Or(x=w237, y=w235) -> (x .or. y?=w238:bool)
                n167 = case shown="True" w238 {
                  tunnel: [string[] ["Forward", "Motor Control", ""] string[] ["Software reset", "Hardware reset", "Motor Control"]] -> w241
                  frame False {
                  }
                  frame True {
                  }
                }
                n168 = Flush Queue(queue=w234) -> ()  [unwired: 1 in, 3 out]
                n169 = Select(t=TLB_MHL_States."Idle" ("Enum"), s=w238, f=TLB_MHL_States."Task 1" ("Enum")) -> (s? t:f=w242:T5)
                n170 = for {
                  shift-right: [w248] -> w239
                  shift-left: w240 -> [w249]
                  tunnel: w241 -> [w247] mode=indexing
                  n171 = Enqueue Element(queue=w249, element=w247) -> (queue out=w248:refnum<queue>)  [unwired: 2 in, 2 out]
                }
              }
              frame "Task 2" {
                # ">>State Logic >>"
                n172 = Flush Queue(queue=w251) -> ()  [unwired: 1 in, 3 out]
                n173 = case shown="True" w254 {
                  tunnel: [w261 string[] ["Hardware reset", "Software reset", "Motor control"]] -> w253
                  tunnel: w252 -> [w260 _]
                  frame False {
                    n174 = case shown="False" w260 {
                      tunnel: [string[] ["Stop", "Ultrasonic read", "Motor Control"] string[] ["Reverse", "Ultrasonic read", "Motor control"]] -> w261
                      frame False {
                      }
                      frame True {
                      }
                    }
                  }
                  frame True {
                  }
                }
                n175 = Select(t=TLB_MHL_States."Idle" ("Enum"), s=w254, f=TLB_MHL_States."Task 2" ("Enum")) -> (s? t:f=w257:T5)
                n176 = for {
                  shift-right: [w266] -> w256
                  shift-left: w255 -> [w267]
                  tunnel: w253 -> [w265] mode=indexing
                  n177 = Enqueue Element(queue=w267, element=w265) -> (queue out=w266:refnum<queue>)  [unwired: 2 in, 2 out]
                }
              }
              frame "Task 3" {
                n178 = Greater Or Equal?(x=w269, y=360.0) -> (x >= y?=w272:bool)
                n179 = Flush Queue(queue=w270) -> ()  [unwired: 1 in, 3 out]
                n180 = Or(x=w272, y=w273) -> (x .or. y?=w274:bool)
                n181 = case shown="False" w274 {
                  tunnel: [string[] ["Rotate CW", "Motor Control"] string[] ["Software reset", "Hardware reset", "Motor Control"]] -> w280
                  frame False {
                  }
                  frame True {
                  }
                }
                n182 = for {
                  shift-right: [w282] -> w278
                  shift-left: w279 -> [w283]
                  tunnel: w280 -> [w281] mode=indexing
                  n183 = Enqueue Element(queue=w283, element=w281) -> (queue out=w282:refnum<queue>)  [unwired: 2 in, 2 out]
                }
                n184 = Select(t=TLB_MHL_States."Idle" ("Enum"), s=w274, f=TLB_MHL_States."Task 3" ("Enum")) -> (s? t:f=w275:T5)
              }
              frame "Task 4" {
                n185 = Flush Queue(queue=w286) -> ()  [unwired: 1 in, 3 out]
                n186 = case shown="True" w288 {
                  tunnel: [string[] ["Forward", "Ultrasonic read", "Motor Control"] string[] ["Stop", "Hardware reset", "Software reset", "Motor Control"]] -> w289
                  frame False {
                  }
                  frame True {
                  }
                }
                n187 = for {
                  shift-right: [w298] -> w291
                  shift-left: w290 -> [w299]
                  tunnel: w289 -> [w297] mode=indexing
                  n188 = Enqueue Element(queue=w299, element=w297) -> (queue out=w298:refnum<queue>)  [unwired: 2 in, 2 out]
                }
                n189 = Select(t=TLB_MHL_States."Task 4a" ("Enum"), s=w288, f=TLB_MHL_States."Task 4" ("Enum")) -> (s? t:f=w294:T5)
              }
              frame "Task 4a" {
                n190 = Greater Or Equal?(x=w300, y=0.5) -> (x >= y?=w304:bool)
                n191 = Flush Queue(queue=w301) -> ()  [unwired: 1 in, 3 out]
                n192 = case shown="True" w304 {
                  tunnel: [string[] ["Right", "Motor Control"] string[] ["Stop", "Hardware reset", "Software reset", "Motor Control"]] -> w307
                  frame False {
                  }
                  frame True {
                  }
                }
                n193 = for {
                  shift-right: [w314] -> w305
                  shift-left: w306 -> [w315]
                  tunnel: w307 -> [w313] mode=indexing
                  n194 = Enqueue Element(queue=w315, element=w313) -> (queue out=w314:refnum<queue>)  [unwired: 2 in, 2 out]
                }
                n195 = Select(t=TLB_MHL_States."Task 4b" ("Enum"), s=w304, f=TLB_MHL_States."Task 4a" ("Enum")) -> (s? t:f=w308:T5)
              }
              frame "Task 4b" {
                n196 = Flush Queue(queue=w317) -> ()  [unwired: 1 in, 3 out]
                n197 = Greater Or Equal?(x=w316, y=0.75) -> (x >= y?=w319:bool)
                n198 = case shown="False" w319 {
                  tunnel: [string[] ["Forward", "Motor control"] string[] ["Stop", "Hardware reset", "Software reset"]] -> w324
                  frame False {
                  }
                  frame True {
                  }
                }
                n199 = for {
                  shift-right: [w330] -> w322
                  shift-left: w323 -> [w331]
                  tunnel: w324 -> [w329] mode=indexing
                  n200 = Enqueue Element(queue=w331, element=w329) -> (queue out=w330:refnum<queue>)  [unwired: 2 in, 2 out]
                }
                n201 = Select(t=TLB_MHL_States."Task 4c" ("Enum"), s=w319, f=TLB_MHL_States."Task 4b" ("Enum")) -> (s? t:f=w321:T5)
              }
              frame "Task 4c" {
                n202 = Flush Queue(queue=w333) -> ()  [unwired: 1 in, 3 out]
                n203 = Less Or Equal?(x=w332, y=-0.65) -> (x <= y?=w335:bool)
                n204 = case shown="False" w335 {
                  tunnel: [string[] ["Left", "Motor Control"] string[] ["Stop", "Hardware reset", "Software reset", "Motor Control"]] -> w340
                  frame False {
                  }
                  frame True {
                  }
                }
                n205 = for {
                  shift-right: [w346] -> w337
                  shift-left: w338 -> [w347]
                  tunnel: w340 -> [w345] mode=indexing
                  n206 = Enqueue Element(queue=w347, element=w345) -> (queue out=w346:refnum<queue>)  [unwired: 2 in, 2 out]
                }
                n207 = Select(t=TLB_MHL_States."Task 4d" ("Enum"), s=w335, f=TLB_MHL_States."Task 4c" ("Enum")) -> (s? t:f=w339:T5)
              }
              frame "Task 4d" {
                n208 = Flush Queue(queue=w349) -> ()  [unwired: 1 in, 3 out]
                n209 = Or(x=w352, y=w351) -> (x .or. y?=w350:bool)
                n210 = case shown="True" w350 {
                  tunnel: [string[] ["Forward", "Ultrasonic Read", "Motor Control"] string[] ["Stop", "Hardware reset", "Software reset", "Motor Control"]] -> w356
                  frame False {
                  }
                  frame True {
                  }
                }
                n211 = for {
                  shift-right: [w362] -> w354
                  shift-left: w355 -> [w363]
                  tunnel: w356 -> [w361] mode=indexing
                  n212 = Enqueue Element(queue=w363, element=w361) -> (queue out=w362:refnum<queue>)  [unwired: 2 in, 2 out]
                }
                n213 = Select(t=TLB_MHL_States."Idle" ("Enum"), s=w350, f=TLB_MHL_States."Task 4d" ("Enum")) -> (s? t:f=w353:T5)
              }
              frame "Reset" {
                n214 = for {
                  shift-right: [w370] -> w365
                  shift-left: w366 -> [w371]
                  tunnel: string[] ["Software reset", "Hardware reset", "Motor Control"] -> [w369] mode=indexing
                  n215 = Enqueue Element(queue=w371, element=w369) -> (queue out=w370:refnum<queue>)  [unwired: 2 in, 2 out]
                }
              }
              frame "Wall follow mode" {
                n216 = Flush Queue(queue=w373) -> ()  [unwired: 1 in, 3 out]
                n217 = case shown="False" w374 {
                  tunnel: [string[] ["IR Sensor Read", "Calculate", "Forward", "Motor Control"] string[] ["Hardware reset", "Software reset", "Motor Control"]] -> w375
                  frame False {
                  }
                  frame True {
                  }
                }
                n218 = for {
                  shift-right: [w384] -> w377
                  shift-left: w376 -> [w385]
                  tunnel: w375 -> [w383] mode=indexing
                  n219 = Enqueue Element(queue=w385, element=w383) -> (queue out=w384:refnum<queue>)  [unwired: 2 in, 2 out]
                }
                n220 = Select(t=TLB_MHL_States."Idle" ("Enum"), s=w374, f=TLB_MHL_States."Wall follow mode" ("Enum")) -> (s? t:f=w379:T5)
              }
              frame "Autodrive" {
                # ">>>Return to idle event>>>"
                n221 = Flush Queue(queue=w395) -> ()  [unwired: 1 in, 3 out]
                n222 = Boolean To (0,1)(Boolean=w391) -> (0, 1=w393:i16)
                n223 = Boolean To (0,1)(Boolean=w390) -> (0, 1=w392:i16)
                n224 = formula code="int8  out;\nif (detect == 0 && stop == 0)\nout = 0;\n\nelse if (detect == 1 && stop == 0)\nout = 1;\n\nelse if (detect == 0 && stop == 1)\nout = 2;\n\nelse\nout = 0;"("stop"=w393, "detect"=w392) -> ("out"=w386:i8)
                n225 = case shown="0, Default" w386 {
                  tunnel: [string[] ["Forward", "Ultrasonic read"] string[] ["Hardware reset", "Software reset", "Rotate Clockwise", ""] string[] ["Hardware reset", "Software reset", "Motor Control", ""]] -> w389
                  frame 0, Default {
                  }
                  frame 1 {
                  }
                  frame 2 {
                  }
                }
                n226 = call "FGV DBL.vi"("Init/Read/Write State"=States_for_Action_Engine."Write", "Input node"=w386) -> ()  [unwired: 1 in, 2 out]
                n227 = for {
                  shift-right: [w405] -> w397
                  shift-left: w396 -> [w406]
                  tunnel: w389 -> [w404] mode=indexing
                  n228 = Enqueue Element(queue=w406, element=w404) -> (queue out=w405:refnum<queue>)  [unwired: 2 in, 2 out]
                }
                n229 = case shown="2" w386 {
                  tunnel: [TLB_MHL_States."Autodrive" ("Enum") TLB_MHL_States."Autodrive a" ("Enum") TLB_MHL_States."Idle" ("Enum")] -> w388
                  frame 0, Default {
                  }
                  frame 1 {
                  }
                  frame 2 {
                  }
                }
              }
              frame "Acquire image" {
                n230 = Flush Queue(queue=w408) -> ()  [unwired: 1 in, 3 out]
                n231 = case shown="True" w409 {
                  tunnel: [string[] ["Cam Acq"] string[] ["Hardware reset", "Software reset", "Cam Exit", ""]] -> w413
                  frame False {
                  }
                  frame True {
                  }
                }
                n232 = for {
                  shift-right: [w419] -> w411
                  shift-left: w412 -> [w420]
                  tunnel: w413 -> [w418] mode=indexing
                  n233 = Enqueue Element(queue=w420, element=w418) -> (queue out=w419:refnum<queue>)  [unwired: 2 in, 2 out]
                }
                n234 = Select(t=TLB_MHL_States."Idle" ("Enum"), s=w409, f=TLB_MHL_States."Acquire image" ("Enum")) -> (s? t:f=w410:T5)
              }
              frame "Processing" {
              }
              frame "Shutdown" {
                # ">>State Logic >>"
                n235 = for {
                  shift-right: [w429] -> w424
                  shift-left: w425 -> [w430]
                  tunnel: string[] ["Software reset", "Hardware reset", "Motor Control", "Cam Exit", "Pre-Exit", "Exit"] -> [w428] mode=indexing
                  n236 = Enqueue Element(queue=w430, element=w428) -> (queue out=w429:refnum<queue>)  [unwired: 2 in, 2 out]
                }
              }
              frame "None" {
              }
              frame "Autodrive a" {
                n237 = Less Or Equal?(x=w441, y=-1.2) -> (x <= y?=w435:bool)
                n238 = case shown="False" w435 {
                  tunnel: [string[] ["Rotate CW", "Ultrasonic read", ""] string[] ["Stop", "Hardware reset", "Software reset", ""]] -> w442
                  frame False {
                  }
                  frame True {
                  }
                }
                n239 = for {
                  shift-right: [w448] -> w444
                  shift-left: w443 -> [w449]
                  tunnel: w442 -> [w447] mode=indexing
                  n240 = Enqueue Element(queue=w449, element=w447) -> (queue out=w448:refnum<queue>)  [unwired: 2 in, 2 out]
                }
                n241 = Select(t=TLB_MHL_States."Idle" ("Enum"), s=w433, f=TLB_MHL_States."Autodrive" ("Enum")) -> (s? t:f=w436:T5)
                n242 = Select(t=w436, s=w435, f=TLB_MHL_States."Autodrive a" ("Enum")) -> (s? t:f=w438:T5)
              }
            }
          }
        }
        n243 = call "FGV DBL.vi"("Init/Read/Write State"=States_for_Action_Engine."Read") -> ("Output"=→"Output":dbl)  [unwired: 2 in, 1 out]
        n244 = local write "GREEN LED State"(w106) -> ()
        "Decision" <- w101
      }
      n245 = call <vilib>:"NavX Close.vi"("NavX Info In"=w29) -> ()  [unwired: 10 in, 1 out]
      n246 = while {
        shift-right: [w63] -> _
        shift-left: _ -> [w64]
        shift-right: [w62] -> _
        shift-left: _ -> [w61]
        stop <- w70 stop-if-true
        (unwired) TRUE
        # "LED Blinker Loop"
        n247 = case shown="\"BLINK\"" "GREEN LED State" {
          tunnel: [FALSE TRUE w78] -> w66
          tunnel: w64 -> [_ _ w78]
          tunnel: [_ _ w79] -> w63
          frame "OFF", Default {
          }
          frame "ON" {
          }
          frame "BLINK" {
            n248 = Not(x=w78) -> (.not. x?=w79:bool)
          }
        }
        n249 = case shown="\"OFF\", Default" "RED LED State" {
          tunnel: [FALSE TRUE w74] -> w65
          tunnel: [_ _ w75] -> w62
          tunnel: w61 -> [_ _ w74]
          frame "OFF", Default {
          }
          frame "ON" {
          }
          frame "BLINK" {
            n250 = Not(x=w74) -> (.not. x?=w75:bool)
          }
        }
        n251 = local write "Green LED"(w66) -> ()
        n252 = local write "Red LED"(w65) -> ()
        n253 = call "FGV Bool.vi"("Init/Read/Write State"=States_for_Action_Engine."Read") -> ("Output node"=w70:bool)  [unwired: 2 in, 1 out]
        n254 = Wait (ms)(milliseconds to wait=u32 500) -> ()  [unwired: 1 out]
      }
      n255 = call <vilib>:"DIO Close.vi"("DIO Info In"=w4) -> ()  [unwired: 10 in, 1 out]
      n256 = call <vilib>:"DIO Close.vi"("error in (no error)"=w21, "DIO Info In"=w27) -> ()  [unwired: 9 in, 1 out]
      n257 = call <vilib>:"DIO Close.vi"("error in (no error)"=w19, "DIO Info In"=w23) -> ()  [unwired: 9 in, 1 out]
      n258 = call <vilib>:"DIO Close.vi"("error in (no error)"=w9, "DIO Info In"=w14) -> ()  [unwired: 9 in, 1 out]
      n259 = call <vilib>:"DIO Close.vi"("error in (no error)"=w7, "DIO Info In"=w13) -> ()  [unwired: 9 in, 1 out]
      n260 = Merge Errors "Merge Errors"(w54, w53) -> (w35:errorcluster)
      n261 = Merge Errors(w39, w35) -> (w30:errorcluster)
      n262 = Destroy User Event(user event=w57, error in=w30) -> ()  [unwired: 1 out]
      n263 = Destroy User Event(user event=w58, error in=w30) -> ()  [unwired: 1 out]
      n264 = Unregister For Events(event registration refnum=w49, error in=w30) -> ()  [unwired: 1 out]
      n265 = Release Queue(queue=w32, error in (no error)=w30) -> (error out=→"error out":errorcluster)  [unwired: 1 in, 2 out]
      n266 = Release Queue(queue=w48, error in (no error)=w30) -> ()  [unwired: 1 in, 3 out]
    }
    frame #2 {
      (unwired) T15."INIT" ("States")
      n267 = call "New motor Control integrated remodeled state based.vi"() -> ()  [unwired: 3 in, 2 out]
    }
    frame #3 {
    }
  }
